vi "RegisterForEvent.vi"(8 "error in (no error)":errorcluster, 11 "object in":refnum<class "WebBrowser_Mgmt.lvclass">) -> (0 "error out":errorcluster, 1 "Event Registration Refnum":refnum<event-registration>, 2 "event callback refnum":refnum<k27>, 3 "object out":refnum<class "WebBrowser_Mgmt.lvclass">, 4 "user event out":refnum<user-event>)   [LabVIEW 2016, in "WebBrowser_Mgmt.lvclass"]
uses:
  WebBrowser_Mgmt.lvclass
  <vilib>/WebServerConfig/Action.ctl
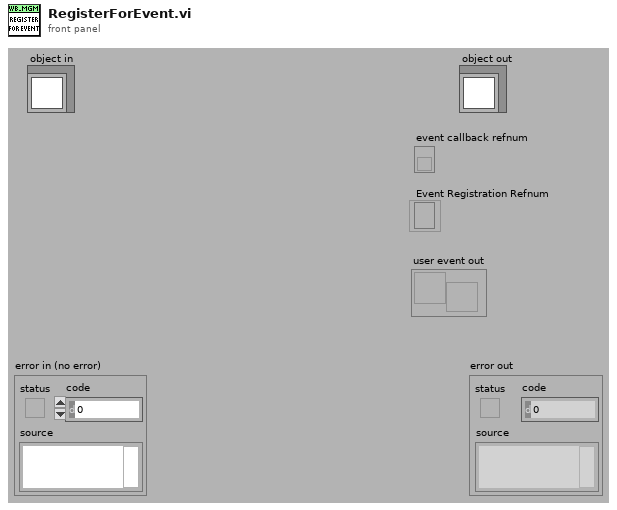
[diagram p1: front panel]
types:
  T1 = typedef "Action.ctl" = cluster{"mimeType":string, "programPath":string}
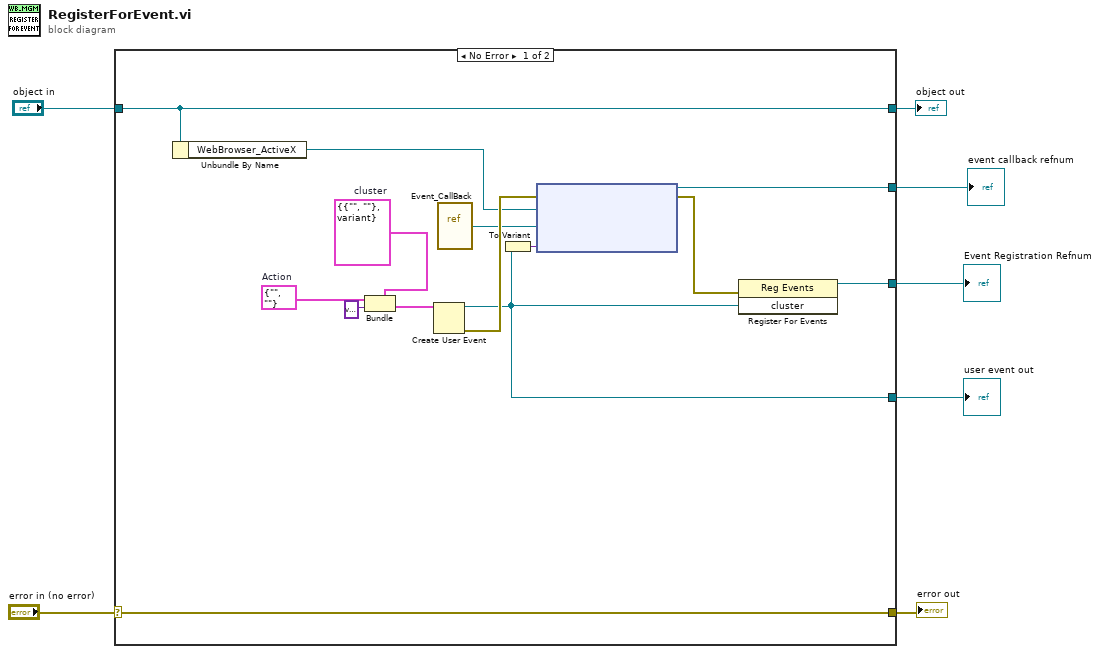
[diagram p0: block diagram]
diagram:
  n1 = case shown="No Error" "error in (no error)" {
    selector: "error in (no error)" -> [w21 w23]
    tunnel: [w21 w23] -> w6
    tunnel: [w20 w22] -> w4
    tunnel: "object in" -> [w20 w22]
    tunnel: [w11 _] -> w3
    tunnel: [w10 _] -> w1
    tunnel: [w9 _] -> w2
    frame No Error {
      w16 = cluster{"Action 2":T1, "Variant":variant} {"Action 2"={"mimeType"="", "programPath"=""}, "Variant"=variant}  # cluster
      w19 = T1 {"mimeType"="", "programPath"=""}  # Action
      n2 = Unbundle By Name(w20) -> ("WebBrowser_ActiveX"=w12:refnum<k7>)
      n3 = Bundle(cluster=w16, "Action 2"=w19, "Variant"=variant) -> (w17:cluster{"Action 2":T1, "Variant":variant})
      n4 = Create User Event(user event datatype=w17) -> (user event=w9:refnum<user-event>, error out=w15:errorcluster)  [unwired: 1 in]
      n5 = vi-ref "Event_CallBack.vi"() -> ("vi reference"=w8:refnum<vi>)
      n6 = To Variant(anything=w9) -> (Variant=w13:variant)
      n7 = node(w15, w12, w8, w13) -> (w11:refnum<k27>, w14:errorcluster)  [unwired: 1 in]
      n8 = register-events(error in=w14, w9) -> (reference out=w10:refnum<event-registration>)  [unwired: 1 in, 1 out]
    }
    frame Error {
    }
  }
  "error out" <- w6
  "object out" <- w4
  "event callback refnum" <- w3
  "user event out" <- w2
  "Event Registration Refnum" <- w1
